vi "Get Routine Object.vi"(6 "Type of Hexaboard":T1, 7 "Settings":T3=enum."Custom", 8 "error in (no error)":errorcluster, 11 "Routine":T2=enum."Secure Syringe") -> (0 "error out":errorcluster, 3 "Routine out":refnum<class "Routine.lvclass">)   [LabVIEW 2021, in "Routine.lvclass"]
uses:
  Routine.lvclass
  Settings.ctl
  Routine Enum.ctl
  TypeOfHexaboard.ctl
  Dispense/Iterative Dispense/Iterative Dispense.lvclass
  C:/Users/User/Documents/UCSB-CMU-GantryCode/UCSB-Gantry-HEP-main/UCSB-Gantry-HEP-main/Classes/Routine/Routine.lvclass
  Pick and Place/Pick and Place.lvclass
  Pick and Place/Pick and Place Type.ctl
  Pick and Place/Pick and Place.lvclass/Pick and Place.ctl
  Secure Syringe/SecureRelease Syringe.lvclass
  Secure Syringe/SecureRelease Syringe.lvclass/SecureRelease Syringe.ctl
  Projects/Sensor Dispense.lvclass
  Pick and Place/Write Pick and Place Type.vi
  Secure Syringe/Write Type.vi
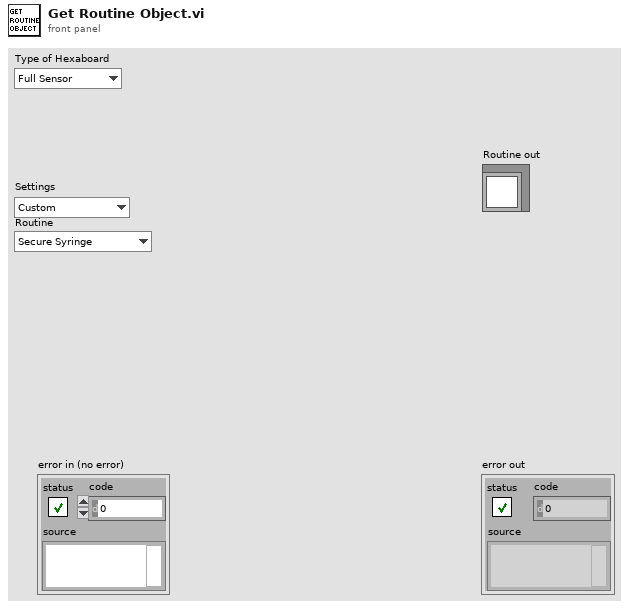
[diagram p1: front panel]
types:
  T1 = typedef "Routine.lvclass/TypeOfHexaboard.ctl" = enum16{"Full Sensor", "Full PCB", "Right Partial PCB", "Right Partial Sensor", "Al Dummy Right Partial Sensor"}
  T2 = typedef "Routine.lvclass/Routine Enum.ctl" = enum16{"Primary Pick Up", "Secondary Pick Up", "Put Down All", "Secure Syringe", "Release Syringe", "Dispense on Plate", "Dispense on Sensor", "Pick Up All", "Put Down Secondary", "Dispense on Kapton", "Full Assembly"}
  T3 = typedef "Routine.lvclass/Settings.ctl" = enum16{"Default", "Custom"}
  T4 = typedef "Pick and Place.lvclass/Pick and Place Type.ctl" = enum16{"Primary Pick Up", "Secondary Pick Up", "Put Down All", "Pick Up All", "Put Down Secondary"}
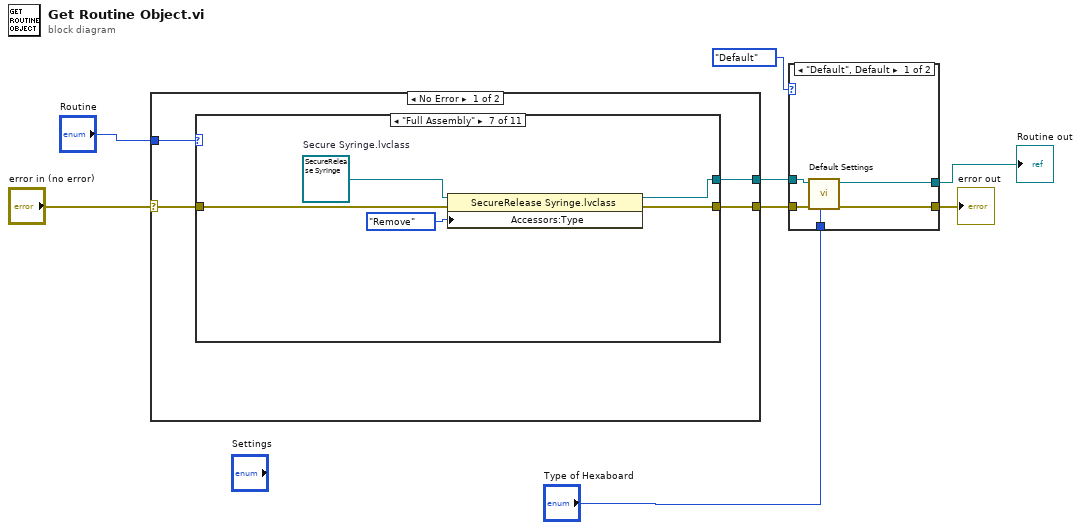
[diagram p0: block diagram]
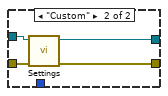
[diagram p2: hidden frame]
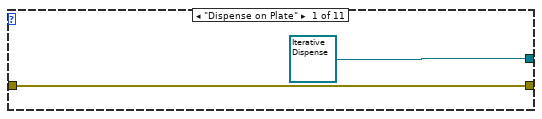
[diagram p3: hidden frame]
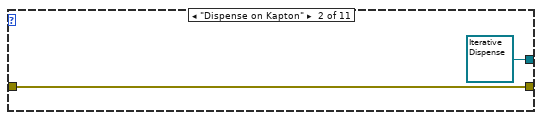
[diagram p4: hidden frame]
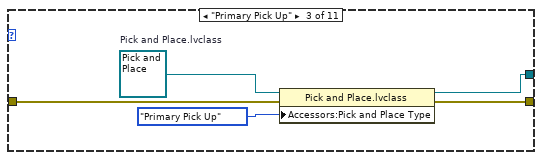
[diagram p5: hidden frame]
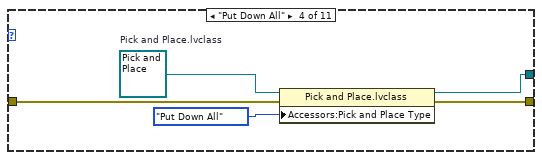
[diagram p6: hidden frame]
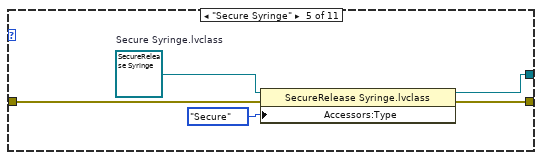
[diagram p7: hidden frame]
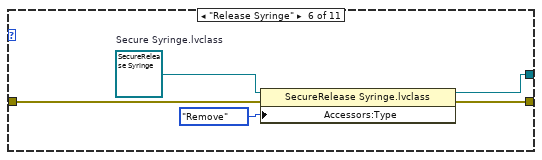
[diagram p8: hidden frame]
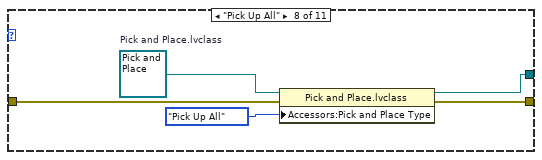
[diagram p9: hidden frame]
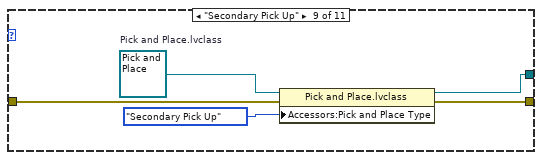
[diagram p10: hidden frame]
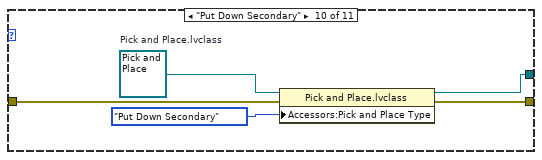
[diagram p11: hidden frame]
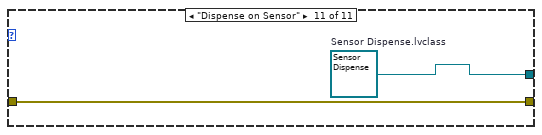
[diagram p12: hidden frame]
diagram:
  n1 = case shown="No Error" "error in (no error)" {
    selector: "error in (no error)" -> [w10 w59]
    tunnel: [w9 w59] -> w3
    tunnel: [w12 _] -> w7
    tunnel: "Routine" -> [w11 _]
    frame No Error {
      n2 = case shown="\"Full Assembly\"" w11 {
        tunnel: [refnum<class "Iterative Dispense.lvclass"> refnum ("Iterative Dispense.lvclass") refnum<class "Iterative Dispense.lvclass"> refnum ("Iterative Dispense.lvclass") w20 w25 w29 w34 w39 w44 w49 w54 w57] -> w12
        tunnel: w10 -> [w14 w16 w18 w23 w28 w33 w38 w43 w48 w53 w58]
        tunnel: [w14 w16 w17 w22 w27 w32 w37 w42 w47 w52 w58] -> w9
        frame "Dispense on Plate" {
        }
        frame "Dispense on Kapton" {
        }
        frame "Primary Pick Up" {
          w21 = refnum<class "Pick and Place.lvclass"> refnum  # Pick and Place.lvclass
          n3 = property class="Pick and Place.lvclass"(reference=w21, error in=w18, "Accessors:Pick and Place Type"=Pick_and_Place_Type."Primary Pick Up" ("Pick and Place Type")) -> (reference out=w20:refnum<class "Pick and Place.lvclass">, error out=w17:errorcluster)
        }
        frame "Put Down All" {
          w26 = refnum<class "Pick and Place.lvclass"> refnum  # Pick and Place.lvclass
          n4 = property class="Pick and Place.lvclass"(reference=w26, error in=w23, "Accessors:Pick and Place Type"=Pick_and_Place_Type."Put Down All" ("Pick and Place Type")) -> (reference out=w25:refnum<class "Pick and Place.lvclass">, error out=w22:errorcluster)
        }
        frame "Secure Syringe" {
          w31 = refnum<class "SecureRelease Syringe.lvclass"> refnum  # Secure Syringe.lvclass
          n5 = property class="SecureRelease Syringe.lvclass"(reference=w31, error in=w28, "Accessors:Type"=enum16{"Secure", "Remove"}."Secure" ("Type")) -> (reference out=w29:refnum<class "SecureRelease Syringe.lvclass">, error out=w27:errorcluster)
        }
        frame "Release Syringe" {
          w36 = refnum<class "SecureRelease Syringe.lvclass"> refnum  # Secure Syringe.lvclass
          n6 = property class="SecureRelease Syringe.lvclass"(reference=w36, error in=w33, "Accessors:Type"=enum16{"Secure", "Remove"}."Remove" ("Type")) -> (reference out=w34:refnum<class "SecureRelease Syringe.lvclass">, error out=w32:errorcluster)
        }
        frame "Full Assembly" {
          w41 = refnum<class "SecureRelease Syringe.lvclass"> refnum  # Secure Syringe.lvclass
          n7 = property class="SecureRelease Syringe.lvclass"(reference=w41, error in=w38, "Accessors:Type"=enum16{"Secure", "Remove"}."Remove" ("Type")) -> (reference out=w39:refnum<class "SecureRelease Syringe.lvclass">, error out=w37:errorcluster)
        }
        frame "Pick Up All" {
          w46 = refnum<class "Pick and Place.lvclass"> refnum  # Pick and Place.lvclass
          n8 = property class="Pick and Place.lvclass"(reference=w46, error in=w43, "Accessors:Pick and Place Type"=Pick_and_Place_Type."Pick Up All" ("Pick and Place Type")) -> (reference out=w44:refnum<class "Pick and Place.lvclass">, error out=w42:errorcluster)
        }
        frame "Secondary Pick Up" {
          w51 = refnum<class "Pick and Place.lvclass"> refnum  # Pick and Place.lvclass
          n9 = property class="Pick and Place.lvclass"(reference=w51, error in=w48, "Accessors:Pick and Place Type"=Pick_and_Place_Type."Secondary Pick Up" ("Pick and Place Type")) -> (reference out=w49:refnum<class "Pick and Place.lvclass">, error out=w47:errorcluster)
        }
        frame "Put Down Secondary" {
          w56 = refnum<class "Pick and Place.lvclass"> refnum  # Pick and Place.lvclass
          n10 = property class="Pick and Place.lvclass"(reference=w56, error in=w53, "Accessors:Pick and Place Type"=Pick_and_Place_Type."Put Down Secondary" ("Pick and Place Type")) -> (reference out=w54:refnum<class "Pick and Place.lvclass">, error out=w52:errorcluster)
        }
        frame "Dispense on Sensor" {
          w57 = refnum<class "Sensor Dispense.lvclass"> refnum  # Sensor Dispense.lvclass
        }
      }
    }
    frame Error {
    }
  }
  n11 = case shown="\"Default\", Default" Settings."Default" ("Settings") {
    tunnel: w7 -> [w63 w67]
    tunnel: [w64 w68] -> w6
    tunnel: w3 -> [w62 w66]
    tunnel: [w61 w65] -> w2
    tunnel: "Type of Hexaboard" -> [w60 _]
    frame "Default", Default {
      n12 = call-dynamic "Default Settings.vi"("Type of Hexaboard"=w60, "error in (no error)"=w62, "Routine in"=w63) -> ("error out"=w61:errorcluster, "Routine out"=w64:refnum<class "Routine.lvclass">)  [unwired: 7 in]
    }
    frame "Custom" {
      n13 = call-dynamic "Settings.vi"("error in (no error)"=w66, "Routine in"=w67) -> ("error out"=w65:errorcluster, "Routine out"=w68:refnum<class "Routine.lvclass">)  [unwired: 8 in]
    }
  }
  "error out" <- w2
  "Routine out" <- w6
